vi "Get Max Reps.vi"(0 "SigMan in":refnum<class "SignalManager.lvclass">, 11 "error in (no error)":errorcluster) -> (4 "SigMan out":refnum<class "SignalManager.lvclass">, 8 "max reps":i32, 15 "error out":errorcluster)   [LabVIEW 2015, in "SignalManager.lvclass"]
uses:
  SignalManager.lvclass
  SignalManager.lvclass/SignalManager.ctl
  Channel/Channel.lvclass/Channel.ctl
  Waveforms/File/File.lvclass
  Waveforms/File/File.lvclass/File.ctl
  Waveforms/File/Read nreps.vi
  Channel/Read Waveform.vi
  Waveforms/Waveform/Waveform.lvclass
  Channel/Channel.lvclass
  Koop/KObject Class/KObject.lvclass
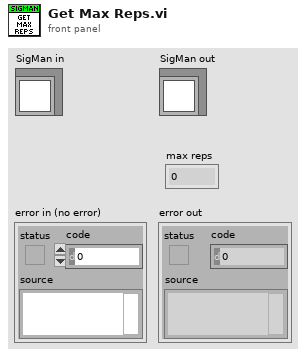
[diagram p1: front panel]
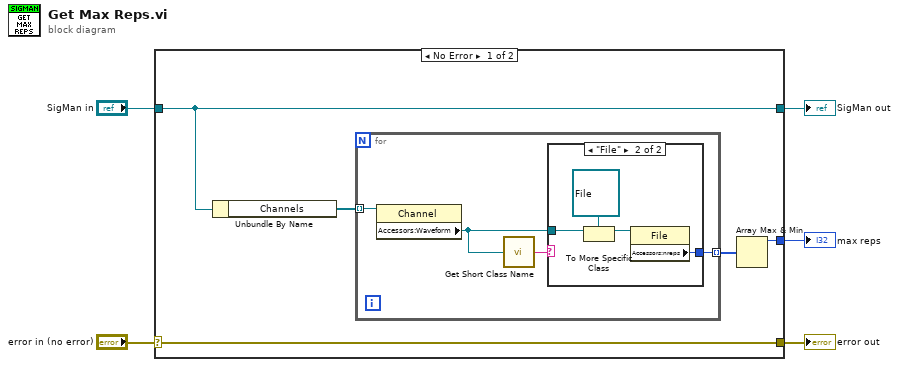
[diagram p0: block diagram]
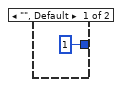
[diagram p2: hidden frame]
diagram:
  n1 = case shown="No Error" "error in (no error)" {
    selector: "error in (no error)" -> [w10 w21]
    tunnel: [w10 w21] -> w4
    tunnel: [w9 w20] -> w2
    tunnel: "SigMan in" -> [w9 w20]
    tunnel: [w6 _] -> w1
    frame No Error {
      n2 = Unbundle By Name(w9) -> ("Channels"=w8:refnum<class "Channel.lvclass">[])
      n3 = for {
        tunnel: w8 -> [w14] mode=indexing
        tunnel: [w11] -> w7 mode=indexing
        n4 = property class="Channel"(reference=w14) -> ("Accessors:Waveform"=w12:refnum<class "Waveform.lvclass">)  [unwired: 1 in, 2 out]
        n5 = call "Get Short Class Name.vi"("KObject in"=w12) -> ("Class"=w13:string)  [unwired: 4 in]
        n6 = case shown="\"File\"" w13 {
          tunnel: w12 -> [_ w19]
          tunnel: [1 ("Accessors:nreps") w16] -> w11
          frame "", Default {
          }
          frame "File" {
            n7 = To More Specific Class(target class=refnum<class "File.lvclass"> refnum ("File"), reference=w19) -> (specific class reference=w17:refnum<class "File.lvclass">)  [unwired: 1 in, 1 out]
            n8 = property class="File"(reference=w17) -> ("Accessors:nreps"=w16:i32)  [unwired: 1 in, 2 out]
          }
        }
      }
      n9 = Array Max & Min(array=w7) -> (max value=w6:i32)  [unwired: 3 out]
    }
    frame Error {
    }
  }
  "error out" <- w4
  "SigMan out" <- w2
  "max reps" <- w1
